vi "ex2.vi"() -> ()   [LabVIEW 2022 SP3]
panel:
  in  "Enum":enum16{"Run", "Reset", "Pause"}(ring)=enum."Reset"
  out "elasped time":dbl
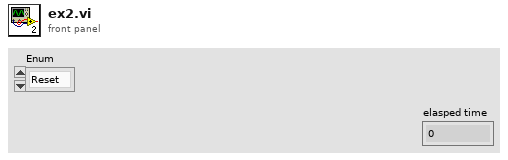
[diagram p1: front panel]
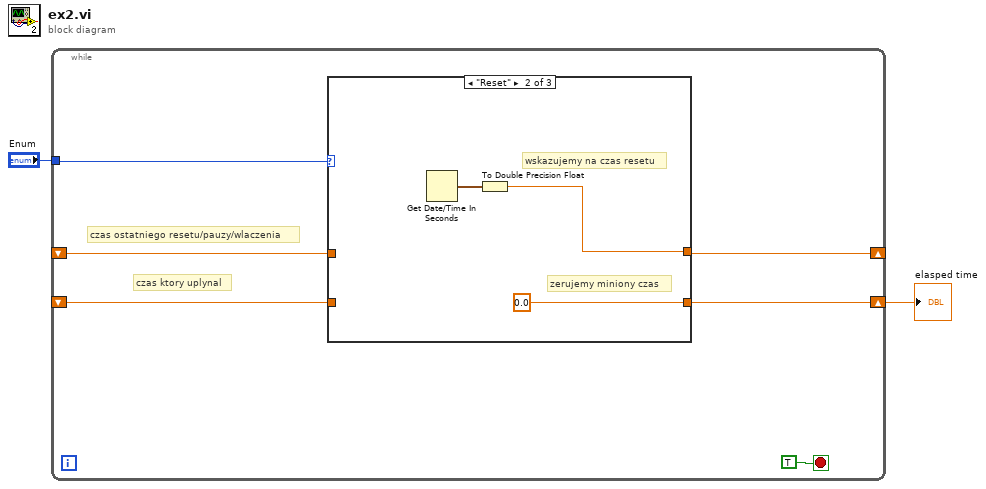
[diagram p0: block diagram]
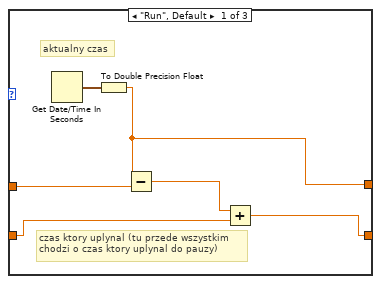
[diagram p2: hidden frame]
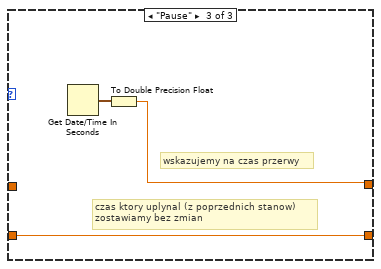
[diagram p3: hidden frame]
diagram:
  n1 = while {
    tunnel: "Enum" -> [w8]
    shift-right: [w7] -> w2
    shift-left: _ -> [w5]
    shift-right: [w4] -> _
    shift-left: _ -> [w3]
    stop <- TRUE stop-if-true
    # "czas ktory uplynal"
    # "czas ostatniego resetu/pauzy/wlaczenia"
    n2 = case shown="\"Reset\"" w8 {
      tunnel: [w9 0.0 w18] -> w7
      tunnel: w5 -> [w11 _ w18]
      tunnel: [w10 w15 w19] -> w4
      tunnel: w3 -> [w13 _ _]
      frame "Run", Default {
        # "czas ktory uplynal (tu przede wszystkim\nchodzi o czas ktory uplynal do pauzy)"
        # "aktualny czas"
        n3 = Get Date/Time In Seconds() -> (seconds since 1Jan1904=w14:timestamp)
        n4 = To Double Precision Float(number=w14) -> (double precision float=w10:dbl)
        n5 = Subtract(x=w10, y=w13) -> (x-y=w12:dbl)
        n6 = Add(x=w12, y=w11) -> (x+y=w9:dbl)
      }
      frame "Reset" {
        # "zerujemy miniony czas"
        # "wskazujemy na czas resetu"
        n7 = Get Date/Time In Seconds() -> (seconds since 1Jan1904=w16:timestamp)
        n8 = To Double Precision Float(number=w16) -> (double precision float=w15:dbl)
      }
      frame "Pause" {
        # "czas ktory uplynal (z poprzednich stanow) \nzostawiamy bez zmian"
        # "wskazujemy na czas przerwy"
        n9 = Get Date/Time In Seconds() -> (seconds since 1Jan1904=w20:timestamp)
        n10 = To Double Precision Float(number=w20) -> (double precision float=w19:dbl)
      }
    }
  }
  "elasped time" <- w2
